vi "logic.vi"() -> ()   [LabVIEW 2020]
panel:
  out "array (last n elements first)":dbl[](array[numeric])
  in  "array":dbl[](array[numeric])
  out "Numeric 2":dbl
  in  "stop":bool
  in  "OK Button":bool
  out "Numeric":dbl
  out "Array":string[](array[string])
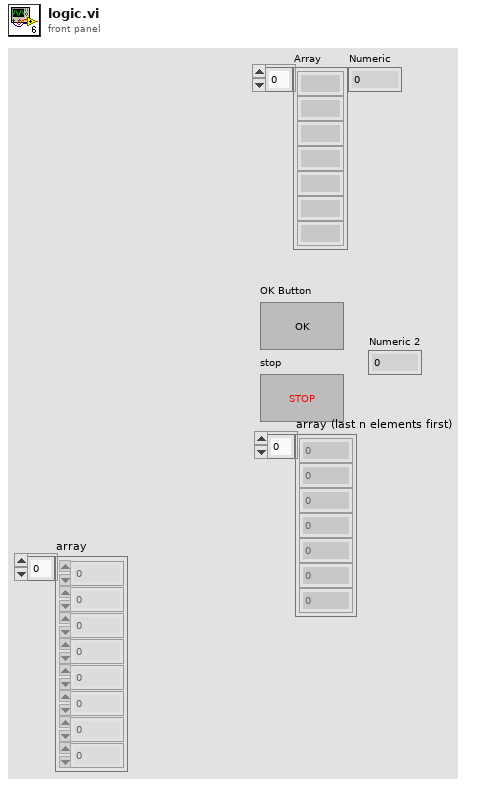
[diagram p1: front panel]
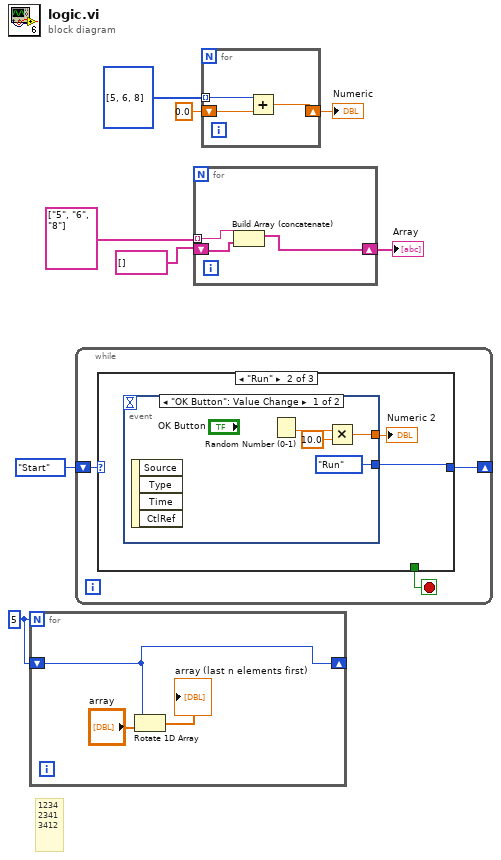
[diagram p0: block diagram]
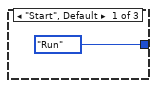
[diagram p2: hidden frame]
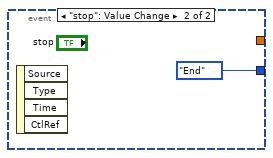
[diagram p3: hidden frame]
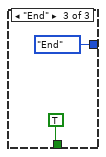
[diagram p4: hidden frame]
diagram:
  w1 = 5
  # "1234\n2341\n3412"
  n1 = for {
    N: w1 -> [_]
    shift-right: [w9] -> _
    shift-left: w1 -> [w9]
    n2 = Rotate 1D Array(1:"array", 2:w9) -> (0:→"array (last n elements first)":dbl[])
  }
  n3 = while {
    shift-right: [w13] -> _
    shift-left: enum16{"Start", "Run", "End"}."Start" -> [w14]
    stop <- w12 stop-if-true
    n4 = case shown="\"Run\"" w14 {
      tunnel: [enum16{"Start", "Run", "End"}."Run" w16 enum16{"Start", "Run", "End"}."End"] -> w13
      tunnel: [_ _ TRUE] -> w12
      frame "Start", Default {
      }
      frame "Run" {
        n5 = event shown="[0] \"OK Button\": Value Change" {
          selector: _ -> [_ _]
          dyn-events: _ -> [_ _]
          timeout: _ -> [_ _]
          tunnel: [w19 _] -> w17
          tunnel: [enum16{"Start", "Run", "End"}."Run" enum16{"Start", "Run", "End"}."End"] -> w16
          event "OK Button": Value Change {
            n6 = event-data() -> ()  [unwired: 1 in, 4 out]
            n7 = Random Number (0-1)() -> (number: 0 to 1=w21:dbl)
            n8 = Multiply(x=w21, y=10.0) -> (x*y=w19:dbl)
          }
          event "stop": Value Change {
            n9 = event-data() -> ()  [unwired: 1 in, 4 out]
          }
        }
        "Numeric 2" <- w17
      }
      frame "End" {
      }
    }
  }
  n10 = for {
    tunnel: string[] ["5", "6", "8"] -> [w27] mode=indexing
    shift-right: [w25] -> w7
    shift-left: string[] [] -> [w26]
    n11 = Build Array (concatenate)(w27, w26) -> (w25:string[])
  }
  "Array" <- w7
  n12 = for {
    shift-right: [w29] -> w4
    shift-left: 0.0 -> [w30]
    tunnel: i32[] [5, 6, 8] -> [w28] mode=indexing
    n13 = Add(x=w28, y=w30) -> (x+y=w29:dbl)
  }
  "Numeric" <- w4
